vi "ODE-VI-21012016.vi"(0 "Param_Value":dbl[](array[numeric])=[0.35, 180.0, 0.3], 1 "Mod_Value":dbl[](array[numeric]), 3 "Param_IDs":string[](array[string])=["k1", "k2", "compartment"], 4 "Mod_IDs":string[](array[string]), 5 "Initial Conditions for  variables":dbl[](array[numeric])=[0.00015, 0.0], 6 "Simulation Parameters":T3={"Time Step"=0.1, "Absolute Tolerance"=1e-07, "Relative Tolerance"=0.0001, "Continuous Solver"=enum."Runge-Kutta 1 (Euler)", "Discrete Time Step"=1.0, "Minimum Time Step"=1e-08, "Maximum Time Step"=1.0, "Initial Time Step"=0.1, "Initial Time"=0.0, "Final Time"=10.0} {"Initial Time Step" min=0.0; "Maximum Time Step" min=0.0; "Minimum Time Step" min=0.0; "Discrete Time Step" min=0.0; "Relative Tolerance" min=0.0; "Absolute Tolerance" min=0.0; "Time Step" min=0.0}, 7 "ODE Right Hand Side":string[](array[string])=["-(compartment*k1*a0)+(compartment*k2*a1^2)", "-2*(compartment*k2*a1^2)+2*(compartment*k1*a0)"], 9 "Del Events":bool, 10 "Event Info":T1, 11 "X (name of variables)":string[](array[string])=["a0", "a1"], 12 "All Variables":string[](array[string]), 13 "Rest_Sp_Init_Amnt":string[](array[string])) -> (14 "Concentration vs. Time":cluster{"times":dbl[], dbl[]}[](graph), 19 "Sim Data":cluster{"times":dbl[], "outputs":dbl[][]} {"outputs" format="%#.9g"})   [LabVIEW 2014]
doc: "This example demonstrates how to use the polymorphic ODE solver in both Formula Sting mode and VI mode. Note that VI mode allows the user to set the values of constants via front panel controls, and the formula is implemented as a call by reference to another VI."
uses:
  <vilib>/Simulation/Implementation/Shared/SIM Continuous Solvers.ctl
  Event Info.ctl
  Stop ODE.vi
  <vilib>/gmath/ode.llb/ODE Solver formula string.vi
  Sim status.vi
  <vilib>/gmath/NI_Gmath.lvlib
panel:
  out "appended array":string[](array[string])
  out "subarray 2":dbl[](array[numeric])
  out "Array":dbl[][](array[numeric])
  out "transposed array":dbl[][](array[numeric])
  out "Assign Val":string[][](array[string])
  out "Assign Var Idx":i32[][](array[numeric])
  out "Var Idx":i32[](array[numeric])
  out "Math Val":string[](array[string])
  out "Math Op":string[](array[string])
  out "outputs":dbl[][](array[numeric])
  out "subarray":dbl[][](array[numeric])
  out "Flag":i32[](array[numeric])
  out "Delay Val Tot":dbl[](array[numeric])
  out "Delay Val":dbl[](array[numeric])
  out "Delay Val":dbl
  out "Priority":dbl[](array[numeric])
  out "Event Idx":i32
  out "Delay":dbl[](array[numeric])
  out "Total Mods":i32
  out "Time":dbl[](array[numeric])
  out "current data size":i32[](array[numeric])
  # "%"
  # "ds1/dt = - (k1*s1 - k2*s2) \nds2/dt = k1*s1 - k2*s2 - (s2*k2^nL/(k2^nL + s3^nL))\nds4/dt = s2*k2^nL/(k2^nL + s3^nL)\nds5/dt = - (s5 * (krp^nRP/(krp^nRP + s4^nRP))*(kG^nG/ (kG^nG + s6^nG)) - k4*s7)\nds7/dt = (s5 * (krp^nRP/(krp^nRP + s4^nRP))*(kG^nG/ (kG^nG + s6^nG)) - k4*s7) - k4*s7\nds8/dt = k4*s7"
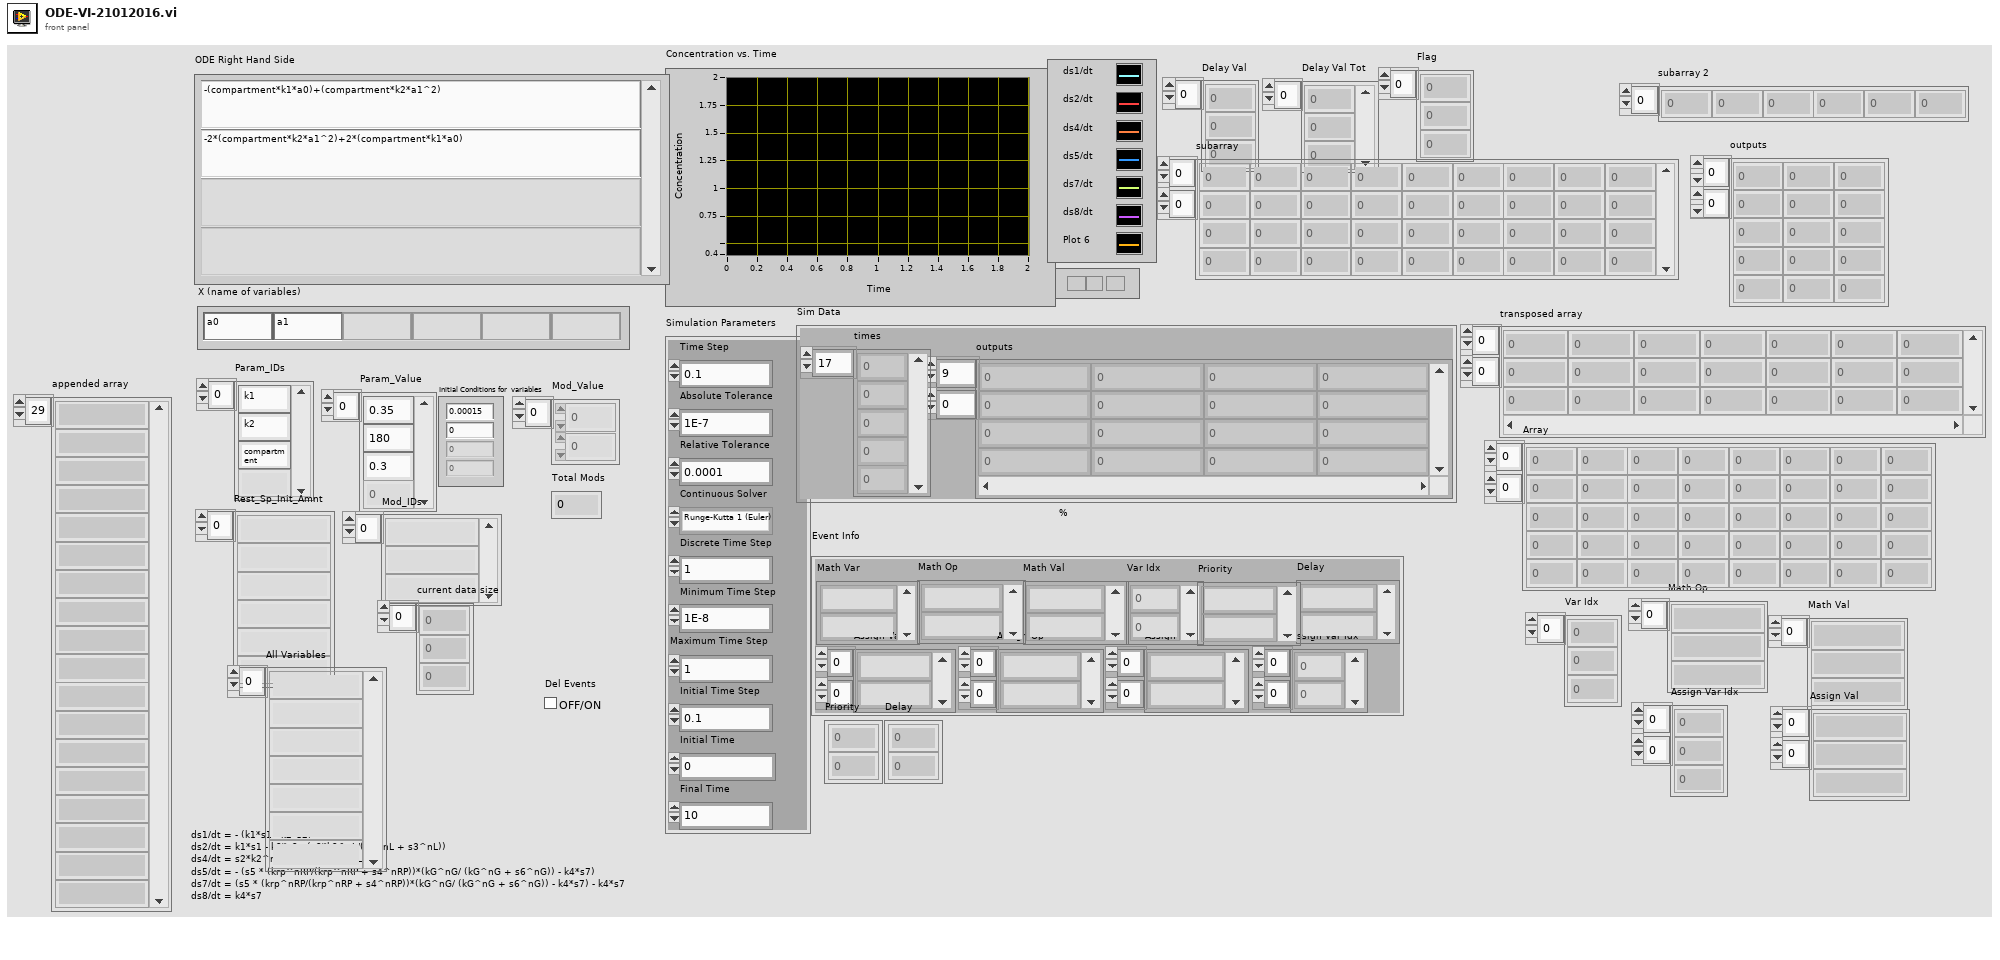
[diagram p1: front panel]
types:
  T1 = typedef "Event Info.ctl" = cluster{"Math Var":string[], "Math Op":string[], "Math Val":string[], "Assign Var":string[][], "Assign Op":string[][], "Assign Val":string[][], "Var Idx":i32[], "Assign Var Idx":i32[][], "Delay":string[], "Priority":string[]}
  T2 = typedef "SIM Continuous Solvers.ctl" = enum16{"Runge-Kutta 1 (Euler)", "Runge-Kutta 2", "Runge-Kutta 3", "Runge-Kutta 4", "Runge-Kutta 23 (variable)", "Runge-Kutta 45 (variable)", "BDF (variable)", "Adams-Moulton (variable)", "Rosenbrock (variable)", "Discrete States Only"}
  T3 = cluster{"Time Step":dbl, "Absolute Tolerance":dbl, "Relative Tolerance":dbl, "Continuous Solver":T2, "Discrete Time Step":dbl, "Minimum Time Step":dbl, "Maximum Time Step":dbl, "Initial Time Step":dbl, "Initial Time":dbl, "Final Time":dbl}
  T4 = cluster{"ODE Right Hand Side":string[], "X (name of variables)":string[], "time":string}
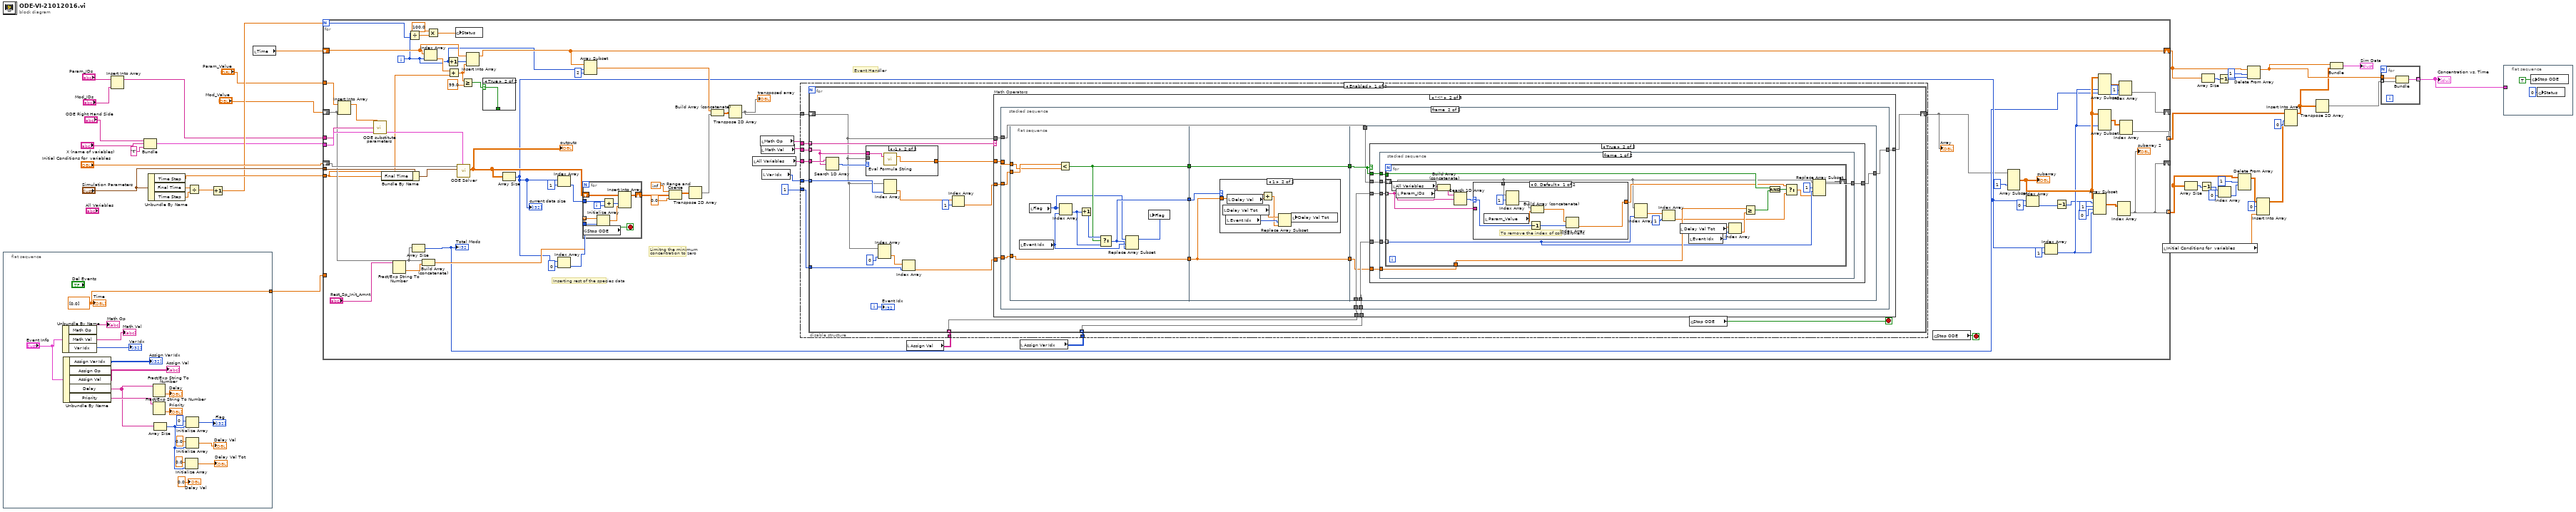
[diagram p0: block diagram]
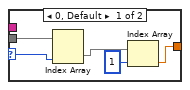
[diagram p3: hidden frame]
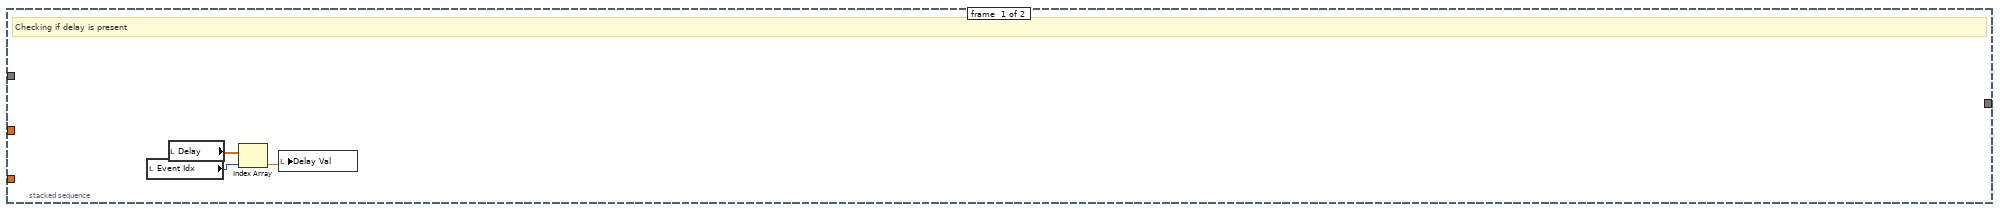
[diagram p5: hidden frame]
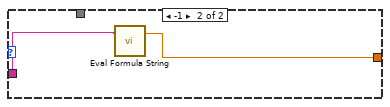
[diagram p8: hidden frame]
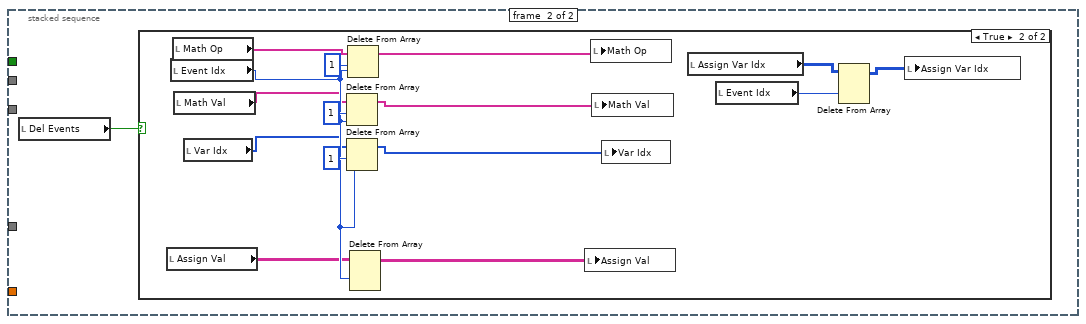
[diagram p9: hidden frame]
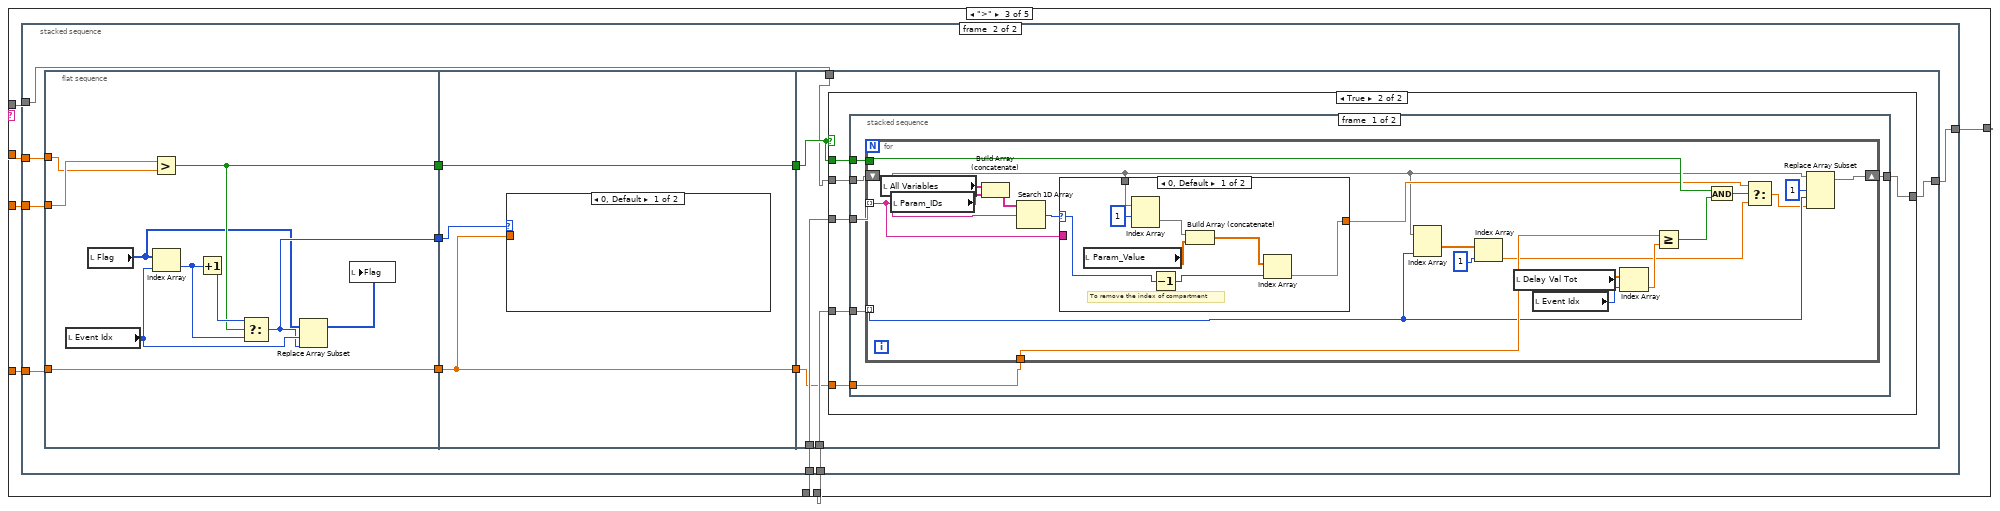
[diagram p11: hidden frame]
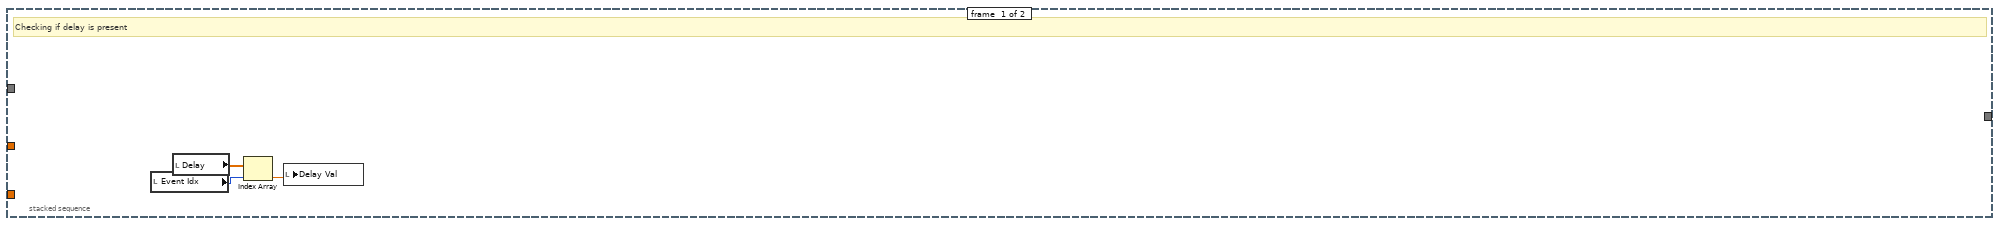
[diagram p12: hidden frame]
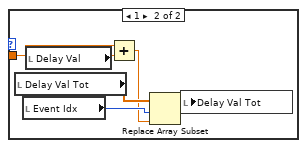
[diagram p13: hidden frame]
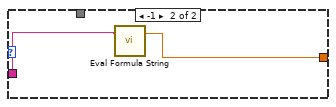
[diagram p15: hidden frame]
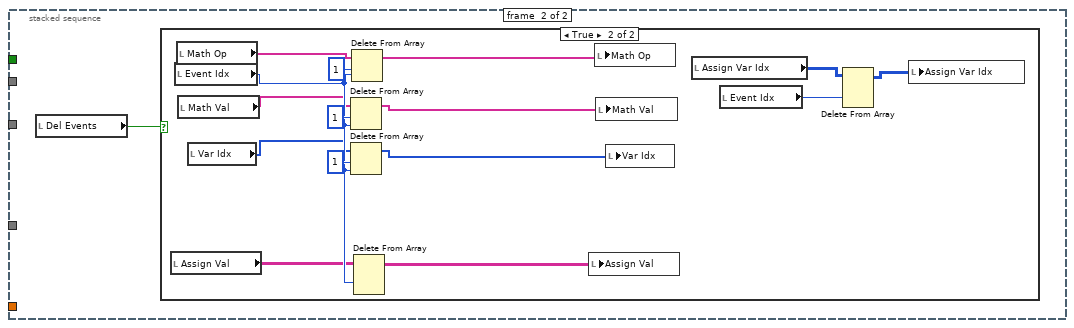
[diagram p16: hidden frame]
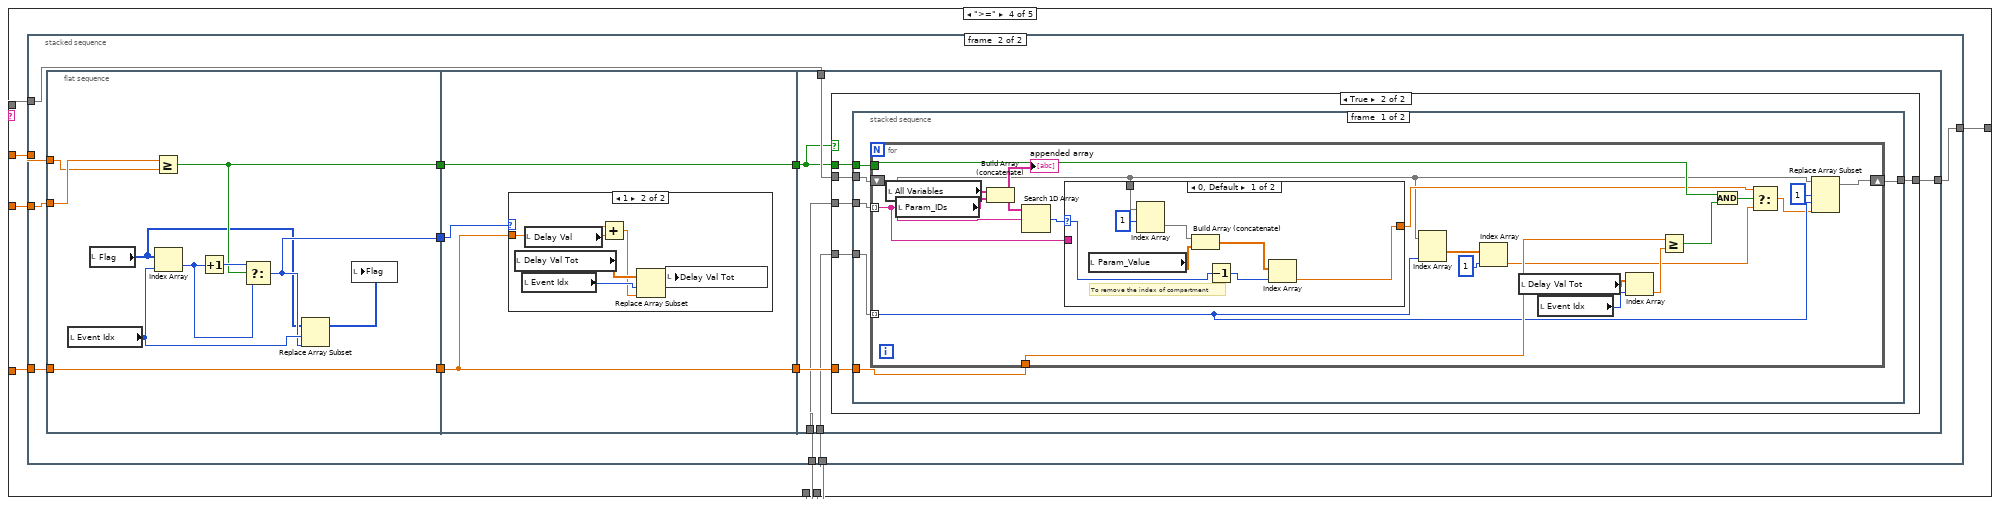
[diagram p18: hidden frame]
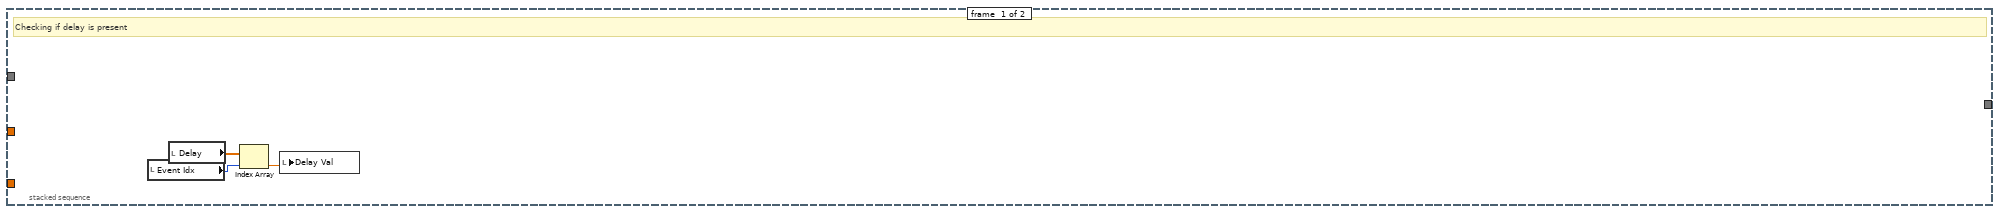
[diagram p19: hidden frame]
diagram:
  n1 = flat-sequence {
    tunnel: [w40] -> w1
    frame #0 {
      w40 = dbl[] [0.0]
      n2 = Unbundle By Name("Event Info") -> ("Math Op"=→"Math Op":string[], "Math Val"=→"Math Val":string[], "Var Idx"=→"Var Idx":i32[])
      n3 = Unbundle By Name("Event Info") -> ("Assign Var Idx"=→"Assign Var Idx":i32[][], "Assign Val"=→"Assign Val":string[][], "Delay"=w49:string[], "Priority"=w52:string[])  [unwired: 1 out]
      n4 = Fract/Exp String To Number(string=w49) -> (number=→"Delay":dbl[])  [unwired: 3 in, 1 out]
      n5 = Fract/Exp String To Number(string=w52) -> (number=→"Priority":dbl[])  [unwired: 3 in, 1 out]
      n6 = Array Size(array=w49) -> (size(s)=w44:i32)
      n7 = Initialize Array(0.0 ("element"), w44) -> (→"Delay Val Tot":dbl[])
      n8 = Initialize Array(0 ("element"), w44) -> (→"Flag":i32[])
      n9 = Initialize Array(0.0 ("element"), w44) -> (→"Delay Val":dbl[])
      "Time" <- w40
      "Delay Val" <- 0.0 ("Delay Val")
    }
  }
  n10 = Insert Into Array(array="Param_IDs", new element="Mod_IDs") -> (w5:string[])  [unwired: 1 in]
  n11 = Bundle("ODE Right Hand Side"="ODE Right Hand Side", "X (name of variables)"="X (name of variables)", "time"="t") -> (w6:T4)  [unwired: 1 in]
  n12 = Unbundle By Name("Simulation Parameters") -> ("Time Step"=w30:dbl, "Final Time"=w32:dbl, "Time Step"=w31:dbl)
  n13 = Divide(x=w32, y=w31) -> (x/y=w28:dbl)
  n14 = Increment(x=w28) -> (x+1=w27:dbl)
  n15 = local read "Time"() -> (w29:dbl[])
  n16 = for {
    N: w27 -> [w72]
    tunnel: "Simulation Parameters" -> [w103]
    shift-right: [w62] -> _
    shift-left: "Initial Conditions for  variables" -> [w124]
    shift-right: [w101] -> w25
    shift-left: w29 -> [w105]
    tunnel: [w62] -> w9 mode=indexing
    tunnel: w30 -> [w82]
    tunnel: [w96] -> w10 mode=indexing
    tunnel: w6 -> [w94]
    tunnel: w5 -> [w93]
    tunnel: "Param_Value" -> [w92]
    shift-right: [w75] -> _
    shift-left: "Mod_Value" -> [w88]
    tunnel: w1 -> [_]
    i -> [w73]
    stop <- w86 stop-if-true
    # "Event Handler"
    # "Limitng the minimum \nconcentration to zero"
    # "Inserting rest of the species data"
    n17 = Insert Into Array(array=w92, new element=w88) -> (w91:dbl[])  [unwired: 1 in]
    n18 = call "ODE substitute parameters.vi"("Formula String Parameters"=w94, "parameters"=w93, "values"=w91) -> ("Formula String Parameters with substitutions"=w95:T4)  [unwired: 2 out]
    n19 = Bundle By Name(cluster=w103, "Final Time"=w82) -> (w102:T3)
    n20 = Fract/Exp String To Number(string="Rest_Sp_Init_Amnt") -> (number=w117:dbl[])  [unwired: 3 in, 1 out]
    n21 = Divide(x=w73, y=w72) -> (x/y=w71:dbl)
    n22 = Array Size(array=w88) -> (size(s)=w87:i32)
    "Total Mods" <- w87
    n23 = Build Array (concatenate)(w88, w117) -> (w116:dbl[])
    n24 = Index Array(array=w105, index=w73) -> (element=w106:dbl)
    n25 = Multiply(x=100.0, y=w71) -> (x*y=w69:dbl)
    n26 = Increment(x=w73) -> (x+1=w104:i32)
    n27 = Add(x=w106, y=w82) -> (x+y=w79:dbl)
    n28 = global write "Sim status.vi" "Status"(w69) -> ()
    n29 = call-poly <vilib>:"ODE Solver.vi"("ODE RHS"=w95, "simulation parameters"=w102, "x0"=w124) -> ("outputs"=w119:dbl[][])  [unwired: 3 in, 5 out]
    "outputs" <- w119
    n30 = Greater Or Equal?(x=w79, y=99.0) -> (x >= y?=w77:bool)
    n31 = Insert Into Array(array=w105, index=w104, new element=w79) -> (w101:dbl[])
    n32 = case shown="True" w77 {
      selector: w77 -> [w125 w126]
      tunnel: [w125 w126] -> _
      frame False {
      }
      frame True {
      }
    }
    n33 = Array Size(array=w119) -> (size(s)=w98:i32[])
    "current data size" <- w98
    n34 = Index Array(array=w98, index=1) -> (element=w122:i32)
    n35 = Index Array(array=w98, index=0) -> (element=w120:i32)
    n36 = for {
      tunnel: w116 -> [w611] mode=indexing
      tunnel: w122 -> [w613]
      tunnel: w120 -> [w610]
      shift-right: [w607] -> w113
      shift-left: w119 -> [w608]
      i -> [w614]
      stop <- w606 stop-if-true
      n37 = global read "Stop ODE.vi" "Stop ODE"() -> (w606:bool)
      n38 = Initialize Array(w611, w610) -> (w609:dbl[])
      n39 = Add(x=w613, y=w614) -> (x+y=w612:i32)
      n40 = Insert Into Array(array=w608, index (col)=w612, new element=w609) -> (w607:dbl[][])  [unwired: 1 in]
    }
    n41 = Array Subset(array=w101, index=w73, length=2) -> (w99:dbl[])
    n42 = In Range and Coerce(upper limit=inf, x=w113, lower limit=0.0) -> (coerced(x)=w84:dbl[][])  [unwired: 1 out]
    n43 = Transpose 2D Array(2D array=w84) -> (transposed array=w83:dbl[][])
    n44 = Build Array (concatenate)(w99, w83) -> (w85:dbl[][])
    n45 = Transpose 2D Array(2D array=w85) -> (transposed array=w81:dbl[][])
    "transposed array" <- w81
    n46 = local read "All Variables"() -> (w63:string[])
    n47 = local read "Math Op"() -> (w68:string[])
    n48 = local read "Math Val"() -> (w67:string[])
    n49 = local read "Var Idx"() -> (w66:i32[])
    n50 = local read "Assign Val"() -> (w64:string[][])
    n51 = local read "Assign Var Idx"() -> (w65:i32[][])
    n52 = disable-structure shown="Enabled" {
      disable-tunnel: w68 -> [w135 w600]
      disable-tunnel: w67 -> [w134 w601]
      disable-tunnel: w66 -> [w133 w602]
      disable-tunnel: w64 -> [w128 w599]
      disable-tunnel: w65 -> [w132 w598]
      disable-tunnel: [w131 w604] -> w61
      disable-tunnel: w81 -> [w130 w605]
      disable-tunnel: 1 ("index") -> [w129 w603]
      disable-tunnel: w63 -> [w127 _]
      frame Enabled {
        n53 = for {
          tunnel: w135 -> [w154] mode=indexing
          tunnel: w134 -> [w138] mode=indexing
          tunnel: w133 -> [w153] mode=indexing
          tunnel: w128 -> [w149] mode=indexing
          tunnel: w132 -> [w152] mode=indexing
          shift-right: [w147] -> w131
          shift-left: w130 -> [w136]
          tunnel: w129 -> [w141]
          tunnel: w127 -> [w139]
          i -> [w150]
          stop <- w151 stop-if-true
          n54 = Search 1D Array(1D array=w139, element=w138) -> (index of element=w137:i32)  [unwired: 1 in]
          n55 = case shown="-1" w137 {
            selector: w137 -> [w158 _]
            tunnel: [w155 w160] -> w148
            tunnel: w138 -> [_ w161]
            tunnel: w136 -> [w159 _]
            frame 0, Default {
              n56 = Index Array(array=w159, index (col)=w158) -> (element=w156:dbl[])  [unwired: 1 in]
              n57 = Index Array(array=w156, index=1) -> (element=w155:dbl)
            }
            frame -1 {
              n58 = call <vilib>:"Eval Formula String.vi"("formula"=w161) -> ("y value"=w160:dbl)  [unwired: 1 in, 1 out]
            }
          }
          n59 = Index Array(array=w136, index (col)=0 ("disabled index (col)")) -> (element=w142:dbl[])  [unwired: 1 in]
          n60 = Index Array(array=w136, index (col)=w153) -> (element=w145:dbl[])  [unwired: 1 in]
          n61 = Index Array(array=w142, index=w141) -> (element=w140:dbl)
          n62 = Index Array(array=w145, index=1) -> (element=w144:dbl)
          n63 = case "Math Operators" shown="\"<\"" w154 {
            tunnel: w148 -> [_ w168 w275 w382 w489]
            tunnel: [w162 w167 w274 w381 w488] -> w147
            tunnel: w136 -> [w162 w169 w276 w383 w490]
            tunnel: w149 -> [_ w166 w273 w380 w487]
            tunnel: w152 -> [_ w165 w272 w379 w486]
            tunnel: w144 -> [_ w164 w271 w377 w485]
            tunnel: w140 -> [_ w163 w270 w378 w484]
            frame "False", Default {
            }
            frame "<" {
              n64 = stacked-sequence {
                tunnel: w168 -> [_ w184]
                tunnel: w169 -> [_ w176]
                tunnel: [_ w175] -> w167
                tunnel: w166 -> [_ w178]
                tunnel: w165 -> [_ w177]
                tunnel: w164 -> [_ w174]
                tunnel: w163 -> [_ w173]
                frame #0 {
                  # "Checking if delay is present"
                  n65 = local read "Event Idx"() -> (w171:i32)
                  n66 = local read "Delay"() -> (w172:dbl[])
                  n67 = Index Array(array=w172, index=w171) -> (element=w170:dbl)
                  n68 = local write "Delay Val"(w170) -> ()
                }
                frame #1 {
                  n69 = flat-sequence {
                    tunnel: w174 -> [w194]
                    tunnel: w184 -> [w193]
                    tunnel: [w188] -> w183
                    tunnel: [w187] -> w182
                    tunnel: [w185] -> w181
                    tunnel: w173 -> [w185]
                    tunnel: w183 -> [w196]
                    tunnel: w182 -> [w197]
                    tunnel: w181 -> [w195]
                    tunnel: [w197] -> w180
                    tunnel: [w195] -> w179
                    tunnel: w180 -> [w209]
                    tunnel: w179 -> [w205]
                    tunnel: w176 -> [w208]
                    tunnel: w177 -> [w206]
                    tunnel: w178 -> [w207]
                    tunnel: [w204] -> w175
                    frame #0 {
                      n70 = local read "Event Idx"() -> (w191:i32)
                      n71 = local read "Flag"() -> (w186:i32[])
                      n72 = Less?(x=w194, y=w193) -> (x < y?=w187:bool)
                      n73 = Index Array(array=w186, index=w191) -> (element=w190:i32)
                      n74 = Increment(x=w190) -> (x+1=w189:i32)
                      n75 = Select(t=w189, s=w187, f=w190) -> (s? t:f=w188:i32)
                      n76 = Replace Array Subset(array=w186, new element=w188, index=w191) -> (w192:i32[])
                      n77 = local write "Flag"(w192) -> ()
                    }
                    frame #1 {
                      n78 = case shown="1" w196 {
                        tunnel: w195 -> [_ w202]
                        frame 0, Default {
                        }
                        frame 1 {
                          n79 = local read "Delay Val Tot"() -> (w201:dbl[])
                          n80 = local read "Event Idx"() -> (w199:i32)
                          n81 = local read "Delay Val"() -> (w203:dbl)
                          n82 = Add(x=w202, y=w203) -> (x+y=w198:dbl)
                          n83 = Replace Array Subset(array=w201, new element=w198, index=w199) -> (w200:dbl[])
                          n84 = local write "Delay Val Tot"(w200) -> ()
                        }
                      }
                    }
                    frame #2 {
                      n85 = case shown="True" w209 {
                        tunnel: w209 -> [_ w216]
                        tunnel: w205 -> [_ w215]
                        tunnel: w208 -> [w210 w214]
                        tunnel: w206 -> [_ w213]
                        tunnel: w207 -> [_ w212]
                        tunnel: [w210 w211] -> w204
                        frame False {
                        }
                        frame True {
                          n86 = stacked-sequence {
                            tunnel: w216 -> [w222 _]
                            tunnel: w215 -> [w221 _]
                            tunnel: w214 -> [w220 _]
                            tunnel: w213 -> [w219 _]
                            tunnel: w212 -> [w218 _]
                            tunnel: [w217 _] -> w211
                            frame #0 {
                              n87 = for {
                                tunnel: w222 -> [w241]
                                tunnel: w221 -> [w240]
                                tunnel: w219 -> [w232] mode=indexing
                                tunnel: w218 -> [w228] mode=indexing
                                shift-right: [w230] -> w217
                                shift-left: w220 -> [w223]
                                n88 = local read "All Variables"() -> (w226:string[])
                                n89 = local read "Param_IDs"() -> (w225:string[])
                                n90 = Build Array (concatenate)(w226, w225) -> (w224:string[])
                                n91 = Search 1D Array(1D array=w224, element=w228) -> (index of element=w229:i32)  [unwired: 1 in]
                                n92 = case shown="0, Default" w229 {
                                selector: w229 -> [w245 _]
                                tunnel: w228 -> [_ w253]
                                tunnel: [w251 w252] -> w227
                                tunnel: w223 -> [w250 _]
                                frame 0, Default {
                                # "To remove the index of compartment"
                                n93 = local read "Param_Value"() -> (w247:dbl[])
                                n94 = Index Array(array=w250, index (row)=1) -> (element=w248:dbl[])  [unwired: 1 in]
                                n95 = Decrement(x=w245) -> (x-1=w244:i32)
                                n96 = Build Array (concatenate)(w248, w247) -> (w246:dbl[])
                                n97 = Index Array(array=w246, index=w244) -> (element=w251:dbl)
                                }
                                frame -1 {
                                n98 = call <vilib>:"Eval Formula String.vi"("formula"=w253) -> ("y value"=w252:dbl)  [unwired: 1 in, 1 out]
                                }
                                }
                                n99 = Index Array(array=w223, index (col)=w232) -> (element=w235:dbl[])  [unwired: 1 in]
                                n100 = Index Array(array=w235, index=1) -> (element=w234:dbl)
                                n101 = local read "Delay Val Tot"() -> (w239:dbl[])
                                n102 = local read "Event Idx"() -> (w238:i32)
                                n103 = Index Array(array=w239, index=w238) -> (element=w237:dbl)
                                n104 = Greater Or Equal?(x=w240, y=w237) -> (x >= y?=w242:bool)
                                n105 = And(x=w241, y=w242) -> (x .and. y?=w243:bool)
                                n106 = Select(t=w227, s=w243, f=w234) -> (s? t:f=w231:dbl)
                                n107 = Replace Array Subset(array=w223, new element=w231, index (row)=1, index (col)=w232) -> (w230:dbl[][])
                              }
                            }
                            frame #1 {
                              n108 = local read "Del Events"() -> (w254:bool)
                              n109 = case shown="True" w254 {
                                frame False {
                                }
                                frame True {
                                n110 = local read "Assign Val"() -> (w259:string[][])
                                n111 = local read "Event Idx"() -> (w266:i32)
                                n112 = local read "Math Op"() -> (w265:string[])
                                n113 = local read "Math Val"() -> (w264:string[])
                                n114 = local read "Var Idx"() -> (w263:i32[])
                                n115 = Delete From Array(array=w264, length=1, index=w266) -> (array with subset deleted=w261:string[])  [unwired: 1 out]
                                n116 = Delete From Array(array=w263, length=1, index=w266) -> (array with subset deleted=w260:i32[])  [unwired: 1 out]
                                n117 = Delete From Array(array=w265, length=1, index=w266) -> (array with subset deleted=w262:string[])  [unwired: 1 out]
                                n118 = Delete From Array(array=w259, index (row)=w266) -> (array with subset deleted=w258:string[][])  [unwired: 2 in, 1 out]
                                n119 = local write "Assign Val"(w258) -> ()
                                n120 = local write "Math Op"(w262) -> ()
                                n121 = local write "Math Val"(w261) -> ()
                                n122 = local write "Var Idx"(w260) -> ()
                                n123 = local read "Assign Var Idx"() -> (w257:i32[][])
                                n124 = local read "Event Idx"() -> (w256:i32)
                                n125 = Delete From Array(array=w257, index (row)=w256) -> (array with subset deleted=w255:i32[][])  [unwired: 2 in, 1 out]
                                n126 = local write "Assign Var Idx"(w255) -> ()
                                }
                              }
                            }
                          }
                        }
                      }
                    }
                  }
                }
              }
            }
            frame ">" {
              n127 = stacked-sequence {
                tunnel: w275 -> [_ w291]
                tunnel: w276 -> [_ w283]
                tunnel: [_ w282] -> w274
                tunnel: w273 -> [_ w285]
                tunnel: w272 -> [_ w284]
                tunnel: w271 -> [_ w281]
                tunnel: w270 -> [_ w280]
                frame #0 {
                  # "Checking if delay is present"
                  n128 = local read "Event Idx"() -> (w278:i32)
                  n129 = local read "Delay"() -> (w279:dbl[])
                  n130 = Index Array(array=w279, index=w278) -> (element=w277:dbl)
                  n131 = local write "Delay Val"(w277) -> ()
                }
                frame #1 {
                  n132 = flat-sequence {
                    tunnel: w281 -> [w301]
                    tunnel: w291 -> [w300]
                    tunnel: w280 -> [w299]
                    tunnel: [w294] -> w290
                    tunnel: [w293] -> w289
                    tunnel: [w299] -> w288
                    tunnel: w290 -> [w303]
                    tunnel: w289 -> [w304]
                    tunnel: w288 -> [w302]
                    tunnel: [w304] -> w287
                    tunnel: [w302] -> w286
                    tunnel: w287 -> [w316]
                    tunnel: w286 -> [w312]
                    tunnel: w283 -> [w315]
                    tunnel: w284 -> [w313]
                    tunnel: w285 -> [w314]
                    tunnel: [w311] -> w282
                    frame #0 {
                      n133 = local read "Event Idx"() -> (w297:i32)
                      n134 = local read "Flag"() -> (w292:i32[])
                      n135 = Greater?(x=w301, y=w300) -> (0:w293:bool)
                      n136 = Index Array(array=w292, index=w297) -> (element=w296:i32)
                      n137 = Increment(x=w296) -> (x+1=w295:i32)
                      n138 = Select(t=w295, s=w293, f=w296) -> (s? t:f=w294:i32)
                      n139 = Replace Array Subset(array=w292, new element=w294, index=w297) -> (w298:i32[])
                      n140 = local write "Flag"(w298) -> ()
                    }
                    frame #1 {
                      n141 = case shown="0, Default" w303 {
                        tunnel: w302 -> [_ w309]
                        frame 0, Default {
                        }
                        frame 1 {
                          n142 = local read "Delay Val Tot"() -> (w308:dbl[])
                          n143 = local read "Event Idx"() -> (w306:i32)
                          n144 = local read "Delay Val"() -> (w310:dbl)
                          n145 = Add(x=w309, y=w310) -> (x+y=w305:dbl)
                          n146 = Replace Array Subset(array=w308, new element=w305, index=w306) -> (w307:dbl[])
                          n147 = local write "Delay Val Tot"(w307) -> ()
                        }
                      }
                    }
                    frame #2 {
                      n148 = case shown="True" w316 {
                        tunnel: w316 -> [_ w323]
                        tunnel: w312 -> [_ w322]
                        tunnel: w315 -> [w317 w321]
                        tunnel: w313 -> [_ w320]
                        tunnel: w314 -> [_ w319]
                        tunnel: [w317 w318] -> w311
                        frame False {
                        }
                        frame True {
                          n149 = stacked-sequence {
                            tunnel: w323 -> [w327 _]
                            tunnel: w322 -> [w324 _]
                            tunnel: w321 -> [w326 _]
                            tunnel: w320 -> [w328 _]
                            tunnel: w319 -> [w325 _]
                            tunnel: [w329 _] -> w318
                            frame #0 {
                              n150 = for {
                                tunnel: w327 -> [w348]
                                tunnel: w324 -> [w347]
                                tunnel: w328 -> [w339] mode=indexing
                                tunnel: w325 -> [w335] mode=indexing
                                shift-right: [w337] -> w329
                                shift-left: w326 -> [w330]
                                n151 = local read "All Variables"() -> (w333:string[])
                                n152 = local read "Param_IDs"() -> (w332:string[])
                                n153 = Build Array (concatenate)(w333, w332) -> (w331:string[])
                                n154 = Search 1D Array(1D array=w331, element=w335) -> (index of element=w336:i32)  [unwired: 1 in]
                                n155 = case shown="0, Default" w336 {
                                selector: w336 -> [w352 _]
                                tunnel: w335 -> [_ w360]
                                tunnel: [w358 w359] -> w334
                                tunnel: w330 -> [w357 _]
                                frame 0, Default {
                                # "To remove the index of compartment"
                                n156 = local read "Param_Value"() -> (w354:dbl[])
                                n157 = Index Array(array=w357, index (row)=1) -> (element=w355:dbl[])  [unwired: 1 in]
                                n158 = Decrement(x=w352) -> (x-1=w351:i32)
                                n159 = Build Array (concatenate)(w355, w354) -> (w353:dbl[])
                                n160 = Index Array(array=w353, index=w351) -> (element=w358:dbl)
                                }
                                frame -1 {
                                n161 = call <vilib>:"Eval Formula String.vi"("formula"=w360) -> ("y value"=w359:dbl)  [unwired: 1 in, 1 out]
                                }
                                }
                                n162 = Index Array(array=w330, index (col)=w339) -> (element=w342:dbl[])  [unwired: 1 in]
                                n163 = Index Array(array=w342, index=1) -> (element=w341:dbl)
                                n164 = local read "Delay Val Tot"() -> (w346:dbl[])
                                n165 = local read "Event Idx"() -> (w345:i32)
                                n166 = Index Array(array=w346, index=w345) -> (element=w344:dbl)
                                n167 = Greater Or Equal?(x=w347, y=w344) -> (x >= y?=w349:bool)
                                n168 = And(x=w348, y=w349) -> (x .and. y?=w350:bool)
                                n169 = Select(t=w334, s=w350, f=w341) -> (s? t:f=w338:dbl)
                                n170 = Replace Array Subset(array=w330, new element=w338, index (row)=1, index (col)=w339) -> (w337:dbl[][])
                              }
                            }
                            frame #1 {
                              n171 = local read "Del Events"() -> (w361:bool)
                              n172 = case shown="True" w361 {
                                frame False {
                                }
                                frame True {
                                n173 = local read "Assign Val"() -> (w366:string[][])
                                n174 = local read "Event Idx"() -> (w373:i32)
                                n175 = local read "Math Op"() -> (w372:string[])
                                n176 = local read "Math Val"() -> (w371:string[])
                                n177 = local read "Var Idx"() -> (w370:i32[])
                                n178 = Delete From Array(array=w371, length=1, index=w373) -> (array with subset deleted=w368:string[])  [unwired: 1 out]
                                n179 = Delete From Array(array=w370, length=1, index=w373) -> (array with subset deleted=w367:i32[])  [unwired: 1 out]
                                n180 = Delete From Array(array=w372, length=1, index=w373) -> (array with subset deleted=w369:string[])  [unwired: 1 out]
                                n181 = Delete From Array(array=w366, index (row)=w373) -> (array with subset deleted=w365:string[][])  [unwired: 2 in, 1 out]
                                n182 = local write "Assign Val"(w365) -> ()
                                n183 = local write "Math Op"(w369) -> ()
                                n184 = local write "Math Val"(w368) -> ()
                                n185 = local write "Var Idx"(w367) -> ()
                                n186 = local read "Assign Var Idx"() -> (w364:i32[][])
                                n187 = local read "Event Idx"() -> (w363:i32)
                                n188 = Delete From Array(array=w364, index (row)=w363) -> (array with subset deleted=w362:i32[][])  [unwired: 2 in, 1 out]
                                n189 = local write "Assign Var Idx"(w362) -> ()
                                }
                              }
                            }
                          }
                        }
                      }
                    }
                  }
                }
              }
            }
            frame ">=" {
              n190 = stacked-sequence {
                tunnel: w382 -> [_ w398]
                tunnel: w383 -> [_ w390]
                tunnel: [_ w389] -> w381
                tunnel: w380 -> [_ w392]
                tunnel: w379 -> [_ w391]
                tunnel: w378 -> [_ w388]
                tunnel: w377 -> [_ w387]
                frame #0 {
                  # "Checking if delay is present"
                  n191 = local read "Event Idx"() -> (w385:i32)
                  n192 = local read "Delay"() -> (w386:dbl[])
                  n193 = Index Array(array=w386, index=w385) -> (element=w384:dbl)
                  n194 = local write "Delay Val"(w384) -> ()
                }
                frame #1 {
                  n195 = flat-sequence {
                    tunnel: w387 -> [w408]
                    tunnel: w398 -> [w407]
                    tunnel: w388 -> [w406]
                    tunnel: [w401] -> w397
                    tunnel: [w400] -> w396
                    tunnel: [w406] -> w395
                    tunnel: w397 -> [w410]
                    tunnel: w396 -> [w411]
                    tunnel: w395 -> [w409]
                    tunnel: [w411] -> w394
                    tunnel: [w409] -> w393
                    tunnel: w394 -> [w418]
                    tunnel: w393 -> [w423]
                    tunnel: w390 -> [w422]
                    tunnel: w391 -> [w421]
                    tunnel: w392 -> [w420]
                    tunnel: [w419] -> w389
                    frame #0 {
                      n196 = local read "Event Idx"() -> (w404:i32)
                      n197 = local read "Flag"() -> (w399:i32[])
                      n198 = Greater Or Equal?(x=w408, y=w407) -> (x >= y?=w400:bool)
                      n199 = Index Array(array=w399, index=w404) -> (element=w403:i32)
                      n200 = Increment(x=w403) -> (x+1=w402:i32)
                      n201 = Select(t=w402, s=w400, f=w403) -> (s? t:f=w401:i32)
                      n202 = Replace Array Subset(array=w399, new element=w401, index=w404) -> (w405:i32[])
                      n203 = local write "Flag"(w405) -> ()
                    }
                    frame #1 {
                      n204 = case shown="1" w410 {
                        tunnel: w409 -> [_ w416]
                        frame 0, Default {
                        }
                        frame 1 {
                          n205 = local read "Delay Val Tot"() -> (w415:dbl[])
                          n206 = local read "Event Idx"() -> (w413:i32)
                          n207 = local read "Delay Val"() -> (w417:dbl)
                          n208 = Add(x=w416, y=w417) -> (x+y=w412:dbl)
                          n209 = Replace Array Subset(array=w415, new element=w412, index=w413) -> (w414:dbl[])
                          n210 = local write "Delay Val Tot"(w414) -> ()
                        }
                      }
                    }
                    frame #2 {
                      n211 = case shown="True" w418 {
                        tunnel: w418 -> [_ w430]
                        tunnel: w423 -> [_ w429]
                        tunnel: w422 -> [w424 w428]
                        tunnel: w421 -> [_ w427]
                        tunnel: w420 -> [_ w426]
                        tunnel: [w424 w425] -> w419
                        frame False {
                        }
                        frame True {
                          n212 = stacked-sequence {
                            tunnel: w430 -> [w435 _]
                            tunnel: w429 -> [w432 _]
                            tunnel: w428 -> [w436 _]
                            tunnel: w427 -> [w433 _]
                            tunnel: w426 -> [w434 _]
                            tunnel: [w431 _] -> w425
                            frame #0 {
                              n213 = for {
                                tunnel: w435 -> [w455]
                                tunnel: w432 -> [w454]
                                tunnel: w433 -> [w446] mode=indexing
                                tunnel: w434 -> [w442] mode=indexing
                                shift-right: [w444] -> w431
                                shift-left: w436 -> [w437]
                                n214 = local read "All Variables"() -> (w440:string[])
                                n215 = local read "Param_IDs"() -> (w439:string[])
                                n216 = Build Array (concatenate)(w440, w439) -> (w438:string[])
                                "appended array" <- w438
                                n217 = Search 1D Array(1D array=w438, element=w442) -> (index of element=w443:i32)  [unwired: 1 in]
                                n218 = case shown="0, Default" w443 {
                                selector: w443 -> [w459 _]
                                tunnel: w442 -> [_ w467]
                                tunnel: [w465 w466] -> w441
                                tunnel: w437 -> [w464 _]
                                frame 0, Default {
                                # "To remove the index of compartment"
                                n219 = local read "Param_Value"() -> (w461:dbl[])
                                n220 = Index Array(array=w464, index (row)=1) -> (element=w462:dbl[])  [unwired: 1 in]
                                n221 = Build Array (concatenate)(w462, w461) -> (w460:dbl[])
                                n222 = Decrement(x=w459) -> (x-1=w458:i32)
                                n223 = Index Array(array=w460, index=w458) -> (element=w465:dbl)
                                }
                                frame -1 {
                                n224 = call <vilib>:"Eval Formula String.vi"("formula"=w467) -> ("y value"=w466:dbl)  [unwired: 1 in, 1 out]
                                }
                                }
                                n225 = Index Array(array=w437, index (col)=w446) -> (element=w449:dbl[])  [unwired: 1 in]
                                n226 = Index Array(array=w449, index=1) -> (element=w448:dbl)
                                n227 = local read "Delay Val Tot"() -> (w453:dbl[])
                                n228 = local read "Event Idx"() -> (w452:i32)
                                n229 = Index Array(array=w453, index=w452) -> (element=w451:dbl)
                                n230 = Greater Or Equal?(x=w454, y=w451) -> (x >= y?=w456:bool)
                                n231 = And(x=w455, y=w456) -> (x .and. y?=w457:bool)
                                n232 = Select(t=w441, s=w457, f=w448) -> (s? t:f=w445:dbl)
                                n233 = Replace Array Subset(array=w437, new element=w445, index (row)=1, index (col)=w446) -> (w444:dbl[][])
                              }
                            }
                            frame #1 {
                              n234 = local read "Del Events"() -> (w468:bool)
                              n235 = case shown="True" w468 {
                                frame False {
                                }
                                frame True {
                                n236 = local read "Assign Val"() -> (w473:string[][])
                                n237 = local read "Event Idx"() -> (w480:i32)
                                n238 = local read "Math Op"() -> (w479:string[])
                                n239 = local read "Math Val"() -> (w478:string[])
                                n240 = local read "Var Idx"() -> (w477:i32[])
                                n241 = Delete From Array(array=w478, length=1, index=w480) -> (array with subset deleted=w475:string[])  [unwired: 1 out]
                                n242 = Delete From Array(array=w477, length=1, index=w480) -> (array with subset deleted=w474:i32[])  [unwired: 1 out]
                                n243 = Delete From Array(array=w479, length=1, index=w480) -> (array with subset deleted=w476:string[])  [unwired: 1 out]
                                n244 = Delete From Array(array=w473, index (row)=w480) -> (array with subset deleted=w472:string[][])  [unwired: 2 in, 1 out]
                                n245 = local write "Assign Val"(w472) -> ()
                                n246 = local write "Math Op"(w476) -> ()
                                n247 = local write "Math Val"(w475) -> ()
                                n248 = local write "Var Idx"(w474) -> ()
                                n249 = local read "Assign Var Idx"() -> (w471:i32[][])
                                n250 = local read "Event Idx"() -> (w470:i32)
                                n251 = Delete From Array(array=w471, index (row)=w470) -> (array with subset deleted=w469:i32[][])  [unwired: 2 in, 1 out]
                                n252 = local write "Assign Var Idx"(w469) -> ()
                                }
                              }
                            }
                          }
                        }
                      }
                    }
                  }
                }
              }
            }
            frame "<=" {
              n253 = stacked-sequence {
                tunnel: w489 -> [_ w505]
                tunnel: w490 -> [_ w497]
                tunnel: [_ w494] -> w488
                tunnel: w487 -> [_ w499]
                tunnel: w486 -> [_ w498]
                tunnel: w485 -> [_ w496]
                tunnel: w484 -> [_ w495]
                frame #0 {
                  # "Checking if delay is present"
                  n254 = local read "Event Idx"() -> (w492:i32)
                  n255 = local read "Delay"() -> (w493:dbl[])
                  n256 = Index Array(array=w493, index=w492) -> (element=w491:dbl)
                  n257 = local write "Delay Val"(w491) -> ()
                }
                frame #1 {
                  n258 = flat-sequence {
                    tunnel: w496 -> [w515]
                    tunnel: w505 -> [w514]
                    tunnel: w495 -> [w513]
                    tunnel: [w508] -> w504
                    tunnel: [w507] -> w503
                    tunnel: [w513] -> w502
                    tunnel: w504 -> [w517]
                    tunnel: w503 -> [w518]
                    tunnel: w502 -> [w516]
                    tunnel: [w518] -> w501
                    tunnel: [w516] -> w500
                    tunnel: w501 -> [w530]
                    tunnel: w500 -> [w526]
                    tunnel: w497 -> [w529]
                    tunnel: w498 -> [w527]
                    tunnel: w499 -> [w528]
                    tunnel: [w525] -> w494
                    frame #0 {
                      n259 = local read "Event Idx"() -> (w511:i32)
                      n260 = local read "Flag"() -> (w506:i32[])
                      n261 = Less Or Equal?(x=w515, y=w514) -> (x <= y?=w507:bool)
                      n262 = Index Array(array=w506, index=w511) -> (element=w510:i32)
                      n263 = Increment(x=w510) -> (x+1=w509:i32)
                      n264 = Select(t=w509, s=w507, f=w510) -> (s? t:f=w508:i32)
                      n265 = Replace Array Subset(array=w506, new element=w508, index=w511) -> (w512:i32[])
                      n266 = local write "Flag"(w512) -> ()
                    }
                    frame #1 {
                      n267 = case shown="1" w517 {
                        tunnel: w516 -> [_ w523]
                        frame 0, Default {
                        }
                        frame 1 {
                          n268 = local read "Delay Val Tot"() -> (w522:dbl[])
                          n269 = local read "Event Idx"() -> (w520:i32)
                          n270 = local read "Delay Val"() -> (w524:dbl)
                          n271 = Add(x=w523, y=w524) -> (x+y=w519:dbl)
                          n272 = Replace Array Subset(array=w522, new element=w519, index=w520) -> (w521:dbl[])
                          n273 = local write "Delay Val Tot"(w521) -> ()
                        }
                      }
                    }
                    frame #2 {
                      n274 = case shown="True" w530 {
                        tunnel: w530 -> [_ w537]
                        tunnel: w526 -> [_ w536]
                        tunnel: w529 -> [w531 w535]
                        tunnel: w527 -> [_ w534]
                        tunnel: w528 -> [_ w533]
                        tunnel: [w531 w532] -> w525
                        frame False {
                        }
                        frame True {
                          n275 = stacked-sequence {
                            tunnel: w537 -> [w543 _]
                            tunnel: w536 -> [w539 _]
                            tunnel: w535 -> [w542 _]
                            tunnel: w534 -> [w540 _]
                            tunnel: w533 -> [w541 _]
                            tunnel: [w538 _] -> w532
                            frame #0 {
                              n276 = for {
                                tunnel: w543 -> [w562]
                                tunnel: w539 -> [w561]
                                tunnel: w540 -> [w553] mode=indexing
                                tunnel: w541 -> [w549] mode=indexing
                                shift-right: [w551] -> w538
                                shift-left: w542 -> [w544]
                                n277 = local read "All Variables"() -> (w547:string[])
                                n278 = local read "Param_IDs"() -> (w546:string[])
                                n279 = Build Array (concatenate)(w547, w546) -> (w545:string[])
                                n280 = Search 1D Array(1D array=w545, element=w549) -> (index of element=w550:i32)  [unwired: 1 in]
                                n281 = case shown="0, Default" w550 {
                                selector: w550 -> [w566 _]
                                tunnel: w549 -> [_ w574]
                                tunnel: [w572 w573] -> w548
                                tunnel: w544 -> [w571 _]
                                frame 0, Default {
                                # "To remove the index of compartment"
                                n282 = local read "Param_Value"() -> (w568:dbl[])
                                n283 = Index Array(array=w571, index (row)=1) -> (element=w569:dbl[])  [unwired: 1 in]
                                n284 = Decrement(x=w566) -> (x-1=w565:i32)
                                n285 = Build Array (concatenate)(w569, w568) -> (w567:dbl[])
                                n286 = Index Array(array=w567, index=w565) -> (element=w572:dbl)
                                }
                                frame -1 {
                                n287 = call <vilib>:"Eval Formula String.vi"("formula"=w574) -> ("y value"=w573:dbl)  [unwired: 1 in, 1 out]
                                }
                                }
                                n288 = Index Array(array=w544, index (col)=w553) -> (element=w556:dbl[])  [unwired: 1 in]
                                n289 = Index Array(array=w556, index=1) -> (element=w555:dbl)
                                n290 = local read "Delay Val Tot"() -> (w560:dbl[])
                                n291 = local read "Event Idx"() -> (w559:i32)
                                n292 = Index Array(array=w560, index=w559) -> (element=w558:dbl)
                                n293 = Greater Or Equal?(x=w561, y=w558) -> (x >= y?=w563:bool)
                                n294 = And(x=w562, y=w563) -> (x .and. y?=w564:bool)
                                n295 = Select(t=w548, s=w564, f=w555) -> (s? t:f=w552:dbl)
                                n296 = Replace Array Subset(array=w544, new element=w552, index (row)=1, index (col)=w553) -> (w551:dbl[][])
                              }
                            }
                            frame #1 {
                              n297 = local read "Del Events"() -> (w575:bool)
                              n298 = case shown="True" w575 {
                                frame False {
                                }
                                frame True {
                                n299 = local read "Assign Val"() -> (w580:string[][])
                                n300 = local read "Event Idx"() -> (w587:i32)
                                n301 = local read "Math Op"() -> (w586:string[])
                                n302 = local read "Math Val"() -> (w585:string[])
                                n303 = local read "Var Idx"() -> (w584:i32[])
                                n304 = Delete From Array(array=w585, length=1, index=w587) -> (array with subset deleted=w582:string[])  [unwired: 1 out]
                                n305 = Delete From Array(array=w584, length=1, index=w587) -> (array with subset deleted=w581:i32[])  [unwired: 1 out]
                                n306 = Delete From Array(array=w586, length=1, index=w587) -> (array with subset deleted=w583:string[])  [unwired: 1 out]
                                n307 = Delete From Array(array=w580, index (row)=w587) -> (array with subset deleted=w579:string[][])  [unwired: 2 in, 1 out]
                                n308 = local write "Assign Val"(w579) -> ()
                                n309 = local write "Math Op"(w583) -> ()
                                n310 = local write "Math Val"(w582) -> ()
                                n311 = local write "Var Idx"(w581) -> ()
                                n312 = local read "Assign Var Idx"() -> (w578:i32[][])
                                n313 = local read "Event Idx"() -> (w577:i32)
                                n314 = Delete From Array(array=w578, index (row)=w577) -> (array with subset deleted=w576:i32[][])  [unwired: 2 in, 1 out]
                                n315 = local write "Assign Var Idx"(w576) -> ()
                                }
                              }
                            }
                          }
                        }
                      }
                    }
                  }
                }
              }
            }
          }
          n316 = global read "Stop ODE.vi" "Stop ODE"() -> (w151:bool)
          "Event Idx" <- w150
        }
      }
      frame Disabled {
        n317 = local read "Delay Val Tot"() -> (w593:dbl[])
        n318 = local read "Delay"() -> (w595:dbl[])
        n319 = local read "Flag"() -> (w594:i32[])
        n320 = local read "Delay Val"() -> (w596:dbl)
        n321 = local read "Priority"() -> (w597:dbl[])
        n322 = call "SBML Events Handler.vi"("Sim Data w/ time"=w605, "Math Op"=w600, "Math Val"=w601, "Var Idx"=w602, "Idx of Time"=w603, "Assign Val"=w599, "Delay"=w595, "Assign Var Idx"=w598, "Flag"=w594, "Priority"=w597, "Delay Val Tot"=w593, "Delay Val"=w596) -> ("Output Data"=w604:dbl[][], "Flag Out"=w592:i32[], "Delay Val Tot Out"=w591:dbl[])  [unwired: 5 in]
        n323 = local write "Delay Val Tot"(w591) -> ()
        n324 = local write "Flag"(w592) -> ()
      }
    }
    "Array" <- w61
    n325 = global read "Stop ODE.vi" "Stop ODE"() -> (w86:bool)
    n326 = Array Subset(array=w61, index (col)=1 ("index (row)")) -> (w90:dbl[][])  [unwired: 3 in]
    "subarray" <- w90
    n327 = Index Array(array=w98, index=0) -> (element=w59:i32)
    n328 = Index Array(array=w98, index=1) -> (element=w89:i32)
    n329 = Decrement(x=w59) -> (x-1=w60:i32)
    n330 = Array Subset(array=w90, index (row)=w60, length (row)=1 ("length"), index (col)=0 ("length"), length (col)=w89) -> (w107:dbl[][])
    n331 = Array Subset(array=w90, index (col)=w89, length (col)=w87) -> (w76:dbl[][])  [unwired: 2 in]
    n332 = Array Subset(array=w90, index (col)=w89) -> (w97:dbl[][])  [unwired: 3 in]
    n333 = Index Array(array=w107) -> (element=w62:dbl[])  [unwired: 2 in]
    "subarray 2" <- w62
    n334 = Index Array(array=w76, index (row)=1) -> (element=w75:dbl[])  [unwired: 1 in]
    n335 = Index Array(array=w97) -> (element=w96:dbl[])  [unwired: 2 in]
  }
  n336 = local read "Initial Conditions for  variables"() -> (w20:dbl[])
  n337 = Array Size(array=w9) -> (size(s)=w17:i32[])
  n338 = Decrement(x=w17) -> (x-1=w15:i32[])
  n339 = Array Size(array=w25) -> (size(s)=w23:i32)
  n340 = Decrement(x=w23) -> (x-1=w22:i32)
  n341 = Index Array(array=w15, index=0) -> (element=w13:i32)
  n342 = Delete From Array(array=w9, length=1, index (row)=w13) -> (array with subset deleted=w12:dbl[][])  [unwired: 1 in, 1 out]
  n343 = Delete From Array(array=w25, length=1, index=w22) -> (array with subset deleted=w18:dbl[])  [unwired: 1 out]
  n344 = Insert Into Array(array=w12, index (row)=0, new element=w20) -> (w8:dbl[][])  [unwired: 1 in]
  n345 = Insert Into Array(array=w10, index (col)=0 ("disabled index (col)"), new element=w8) -> (w7:dbl[][])  [unwired: 1 in]
  n346 = Transpose 2D Array(2D array=w7) -> (transposed array=w21:dbl[][])
  n347 = Bundle("Time"=w18, w7) -> (→"Sim Data":cluster{"Time":dbl[], dbl[][]})  [unwired: 1 in]
  n348 = for {
    tunnel: w18 -> [w616]
    tunnel: [w617] -> w2 mode=indexing
    tunnel: w21 -> [w615] mode=indexing
    n349 = Bundle("Time"=w616, w615) -> (w617:cluster{"Time":dbl[], dbl[]})  [unwired: 1 out]
  }
  "Concentration vs. Time" <- w2
  n350 = flat-sequence {
    tunnel: w2 -> [_]
    frame #0 {
      n351 = global write "Stop ODE.vi" "Stop ODE"(TRUE) -> ()
      n352 = global write "Sim status.vi" "Status"(0 ("Status")) -> ()
    }
  }
